vi "bubble_sort.vi"() -> ()   [LabVIEW 2021]
panel:
  out "sorted":dbl[](array[numeric])
  out "unsorted":dbl[](array[numeric])
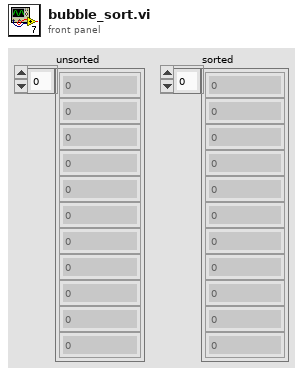
[diagram p1: front panel]
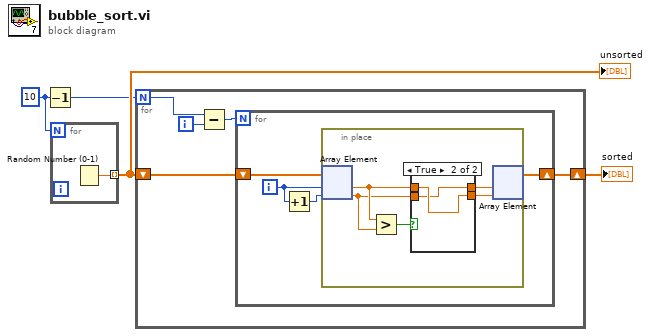
[diagram p0: block diagram]
diagram:
  w3 = 10
  n1 = Decrement(x=w3) -> (x-1=w2:i32)
  n2 = for {
    N: w3 -> [_]
    tunnel: [w5] -> w4 mode=indexing
    n3 = Random Number (0-1)() -> (number: 0 to 1=w5:dbl)
  }
  "unsorted" <- w4
  n4 = for {
    N: w2 -> [w10]
    shift-right: [w6] -> w1
    shift-left: w4 -> [w7]
    i -> [w8]
    n5 = Subtract(x=w10, y=w8) -> (x-y=w9:i32)
    n6 = for {
      N: w9 -> [_]
      shift-right: [w11] -> w6
      shift-left: w7 -> [w14]
      i -> [w13]
      n7 = Increment(x=w13) -> (x+1=w12:i32)
      n8 = in-place {
        n9 = in-place-array #1(w14, w13, w12) -> (w17:dbl, w15:dbl)
        n10 = Greater?(x=w17, y=w15) -> (0:w19:bool)
        n11 = case shown="True" w19 {
          tunnel: [w20 w23] -> w18
          tunnel: w17 -> [w21 w23]
          tunnel: [w21 w22] -> w16
          tunnel: w15 -> [w20 w22]
          frame False {
          }
          frame True {
          }
        }
        n12 = in-place-array #1(w16, w18) -> (w11:dbl[])  [unwired: 2 out]
      }
    }
  }
  "sorted" <- w1
